vi "RVC - Inverse Kinematics for Puma 560.vi"() -> ()   [LabVIEW 2013]
doc: "This example shows how to calculate the joint positions of a PUMA 560 robot as it travels in a straight line trajectory.\n\nRequirements\nLabVIEW Robotics"
uses:
  <vilib>/robotics/Kinematics/Generate Cartesian Trajectory (Int).vi
  <vilib>/robotics/Kinematics/Robot/Inverse Kinematics (Point).vi
  <vilib>/robotics/Kinematics/Robot/Forward Kinematics (Point).vi
  <vilib>/picture/3D Picture Control/Object/Add Object (reference).vi
  <vilib>/robotics/Kinematics/NI_Kinematics.lvlib
  <vilib>/robotics/Kinematics/Plotting/NI_Robotics_3DKinematics.lvlib
  <vilib>/picture/3D Picture Control/NI_3D Picture Control.lvlib
panel:
  out "joint positions":dbl[](array[numeric])
  out "First Run Signal":bool=TRUE
  out "Current Z":dbl=0.4
  out "Current Y":dbl=0.5
  out "Current X":dbl
  in  "End Z":dbl=0.4
  in  "End Y":dbl=0.5
  in  "End X":dbl
  in  "Start Z":dbl
  in  "Start Y":dbl=0.5
  in  "Start X":dbl=0.6
  in  "Number of Trajectory Points":i32=36
  out "error out":errorcluster
  out "3D Picture Control":refnum<vi>(3d-picture)
  in  "stop":bool
  in  "Play":bool
  # "This example shows how to calculate the joint positions of a PUMA 560 robot as it travels in a straight line trajectory.\n\n1) Run the example and observe the motion of the arm\n2) Change the Start or End Position\n3) Press Play to view the new trajectory\n4) If the Start or End Position is not achievable an error will occur."
  # "Start Position"
  # "End Position"
  # "Current Position"
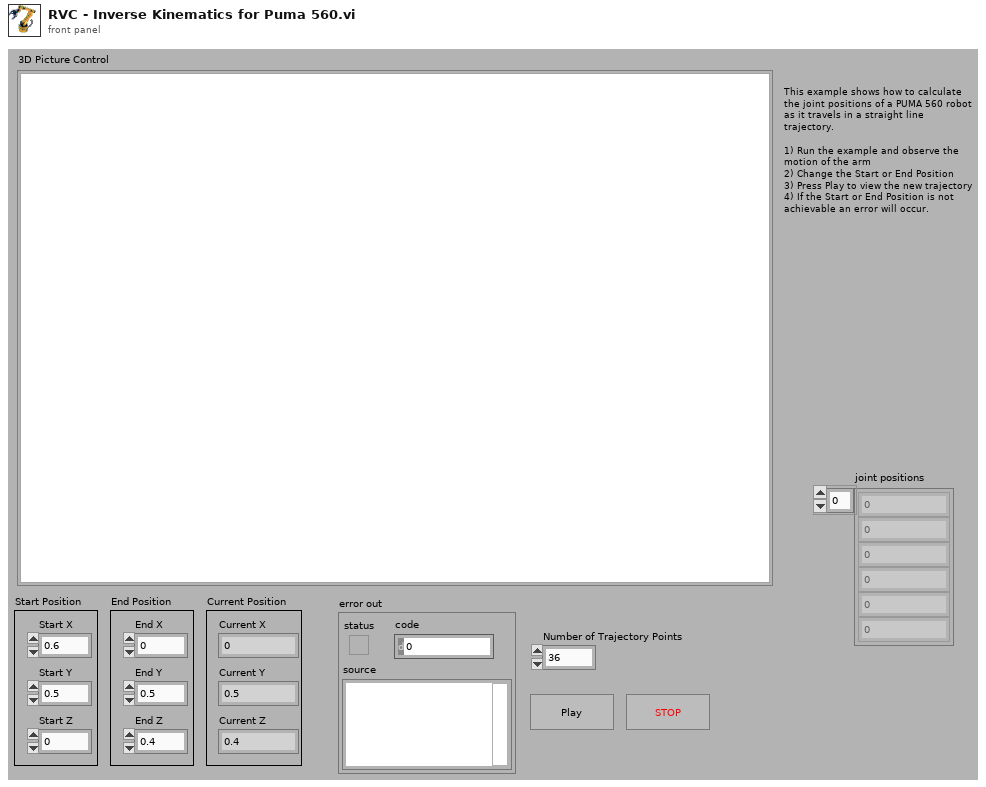
[diagram p1: front panel]
types:
  T1 = typedef "NI_Matrix.lvlib/RealMatrix.ctl" = dbl[][]
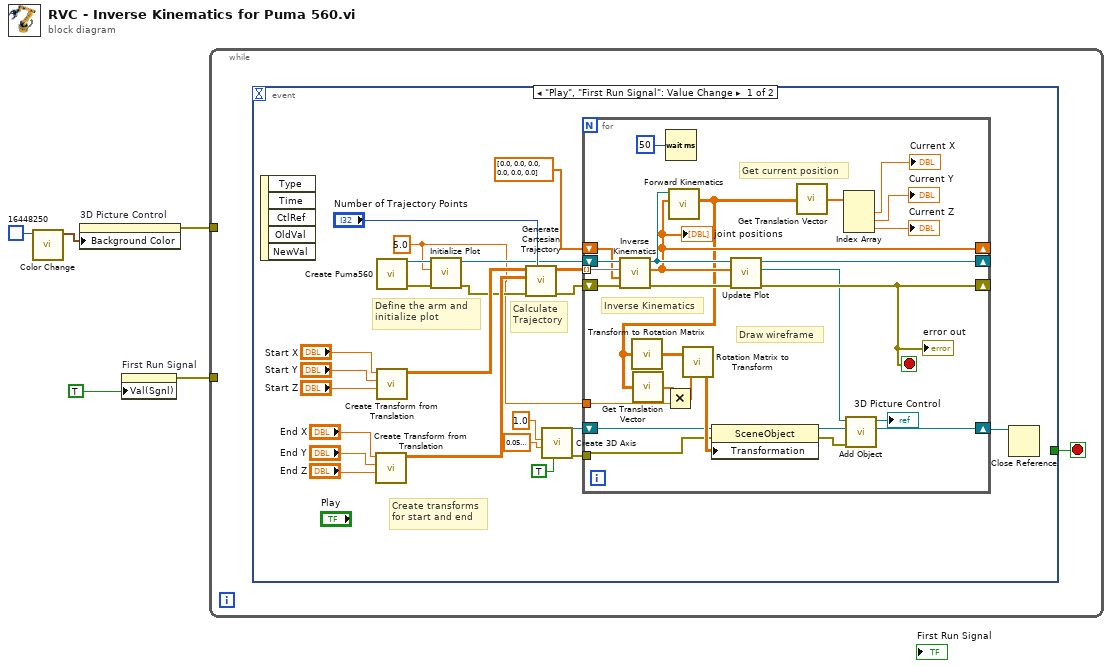
[diagram p0: block diagram]
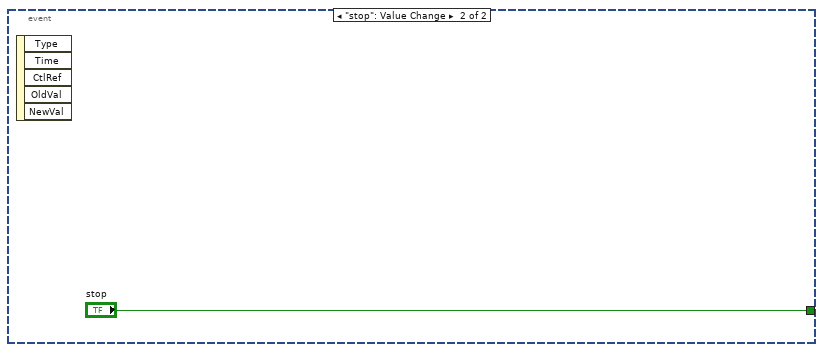
[diagram p2: hidden frame]
diagram:
  n1 = call <vilib>:"Color Change.vi"("Color"=u32 16448250) -> ("RGBA"=w2:cluster{"R":sgl, "G":sgl, "B":sgl, "A":sgl})  [unwired: 10 in]
  n2 = property on="3D Picture Control" class="SceneGraphDisp (strict)"("Background Color"=w2) -> (error out=w3:errorcluster)  [unwired: 2 in, 1 out]
  n3 = property on="First Run Signal" class="Bool (strict)"("Val(Sgnl)"=TRUE ("Value (Signaling)")) -> (error out=w5:errorcluster)  [unwired: 2 in, 1 out]
  n4 = while {
    tunnel: w5 -> [_]
    tunnel: w3 -> [_]
    stop <- w6 stop-if-true
    n5 = event shown="[0] \"Play\", \"First Run Signal\": Value Change" {
      selector: _ -> [_ _]
      dyn-events: _ -> [_ _]
      timeout: _ -> [_ _]
      tunnel: [_ "stop"] -> w6
      event "Play", "First Run Signal": Value Change {
        w13 = 5.0 ("scale (1)")
        # "Calculate \nTrajectory"
        # "Create transforms\nfor start and end"
        # "Define the arm and \ninitialize plot"
        n6 = event-data() -> ()  [unwired: 1 in, 5 out]
        n7 = call <vilib>:"Create Transform from Translation.vi"("z"="End Z", "y"="End Y", "x"="End X") -> ("transform"=w22:T1)  [unwired: 1 in, 7 out]
        n8 = call <vilib>:"Create Puma560.vi"() -> ("error out"=w17:errorcluster, "Puma560 Robot"=w18:refnum<class "NI_Robotics_Serial Robot Arm.lvclass">)  [unwired: 1 in, 9 out]
        n9 = call <vilib>:"Create Transform from Translation.vi"("z"="Start Z", "y"="Start Y", "x"="Start X") -> ("transform"=w23:T1)  [unwired: 1 in, 7 out]
        n10 = call <vilib>:"Initialize Plot.vi"("error in (no error)"=w17, "scale (1)"=w13, "serial arm in"=w18) -> ("error out"=w16:errorcluster, "serial arm out"=w15:refnum<class "NI_Robotics_Serial Robot Arm.lvclass">)  [unwired: 7 in]
        n11 = call-poly <vilib>:"Generate Cartesian Trajectory.vi"("intermediate points"="Number of Trajectory Points", "error in (no error)"=w16, "end transform"=w22, "start transform"=w23) -> ("error out"=w19:errorcluster, "interpolated trajectory"=w20:dbl[][][])  [unwired: 6 in]
        n12 = call <vilib>:"Create 3D Axis.vi"("Axis label?"=TRUE, "Radius"=sgl 0.05, "Length"=sgl 1.0) -> ("error out"=w9:errorcluster, "New Object Refnum"=w10:refnum<vi>)  [unwired: 7 in]
        n13 = for {
          shift-right: [w47] -> _
          shift-left: w19 -> [w52]
          tunnel: w20 -> [w55] mode=indexing
          shift-right: [w44] -> _
          shift-left: w15 -> [w54]
          shift-right: [w45] -> _
          shift-left: dbl[] [0.0, 0.0, 0.0, 0.0, 0.0, 0.0] ("joint positions") -> [w53]
          tunnel: w13 -> [w35]
          tunnel: w9 -> [w31]
          shift-right: [w30] -> w7
          shift-left: w10 -> [w32]
          stop <- w47 stop-if-true
          # "Get current position"
          # "Draw wireframe"
          # "Inverse Kinematics"
          n14 = call-poly <vilib>:"Inverse Kinematics.vi"("error in (no error)"=w52, "current joint positions"=w53, "end effector transform"=w55, "serial arm in"=w54) -> ("error out"=w48:errorcluster, "joint positions"=w45:dbl[], "serial arm out"=w46:refnum<class "NI_Robotics_Serial Robot Arm.lvclass">)  [unwired: 4 in, 1 out]
          "joint positions" <- w45
          n15 = Wait (ms)(milliseconds to wait=50) -> ()  [unwired: 1 out]
          n16 = call-poly <vilib>:"Forward Kinematics.vi"("joint positions"=w45, "serial arm in"=w46) -> ("end effector transform"=w33:T1)  [unwired: 7 in, 2 out]
          n17 = call <vilib>:"Transform to Rotation Matrix.vi"("transform"=w33) -> ("rotation matrix"=w36:T1)
          n18 = call <vilib>:"Get Translation Vector.vi"("transform"=w33) -> ("translation vector"=w38:dbl[])
          n19 = Multiply(x=w38, y=w35) -> (x*y=w37:dbl[])
          n20 = call <vilib>:"Rotation Matrix to Transform.vi"("translation vector"=w37, "rotation matrix"=w36) -> ("transform"=w34:T1)
          n21 = property class="SceneObject"(reference=w32, error in=w31, "Transformation"=w34) -> (reference out=w41:refnum<vi>, error out=w42:errorcluster)
          n22 = call <vilib>:"Update Plot.vi"("error in (no error)"=w48, "joint positions"=w45, "serial arm in"=w46) -> ("error out"=w47:errorcluster, "serial arm scene"=w40:refnum<vi>, "serial arm out"=w44:refnum<class "NI_Robotics_Serial Robot Arm.lvclass">)  [unwired: 6 in]
          "error out" <- w47
          n23 = call <vilib>:"Get Translation Vector.vi"("transform"=w33) -> ("translation vector"=w43:dbl[])
          n24 = Index Array(array=w43) -> (element #1=→"Current X":dbl, element #2=→"Current Y":dbl, element #3=→"Current Z":dbl)  [unwired: 3 in]
          n25 = call-poly <vilib>:"Add Object.vi"("error in (no error)"=w42, "New Object In"=w41, "Scene Object In"=w40) -> ("New Object Out"=w30:refnum<vi>, "Scene Object Out"=→"3D Picture Control":refnum<vi>)  [unwired: 6 in, 1 out]
        }
        n26 = Close Reference(reference=w7) -> ()  [unwired: 1 in, 1 out]
      }
      event "stop": Value Change {
        n27 = event-data() -> ()  [unwired: 1 in, 5 out]
      }
    }
  }
